vi "SetUp_Action.vi"(7 "Slot":T3, 8 "error in":errorcluster, 11 "GuiRef":T1={"StringOut"=refnum, "AbortOnFail"=refnum, "SN"=refnum, "SN_Length"=refnum, "TestResult"=refnum, "CycleTime"=refnum, "ErrorCode"=refnum, "UUTStatus"=refnum, "DataBaseEnable?"=refnum, "DUTModel"=refnum, "FixtureID"=refnum, "OperatorID"=refnum, "SNReady"=refnum, "StopSlot"=refnum, "NextStep"=refnum, "PassYeild"=refnum, "Failed"=refnum, "Passed"=refnum, "Tested"=refnum, "TestItemsCtl"={"StepName"="", "TestEnable"=FALSE, "LoopCount"=0, "StopOnFail"=FALSE, "Index"=0, "TestName"="", "通道"="", "参数"="", "TimeStart"=0}, "ProcessBar"=refnum, "Slot"=enum."Slot1", "Row"=3, "States"=refnum, "TestMode"=refnum, "循环次数-DUT"=refnum, "波形图"=refnum, "产品型号"=refnum, "子面板"=refnum, "测试失败项目"=refnum, "测试结果"=refnum, "DUT"=refnum, "Starttime"=refnum, "SlotReady"=refnum, "版本信息"=refnum, "WIFI_1"=refnum, "WIFI_2"=refnum, "直通率"=refnum, "卡1开卡结果"=refnum, "卡2开卡结果"=refnum}) -> (0 "error out":errorcluster, 3 "ScanSNOK":bool)   [LabVIEW 2013]
uses:
  SystemCode/SysControl/Slot.ctl
  SystemCode/SysControl/Reference.ctl
  SystemCode/SysControl/TestItemsCTL.ctl
  SystemCode/SysControl/LEDState.ctl
  GlobalValue.vi
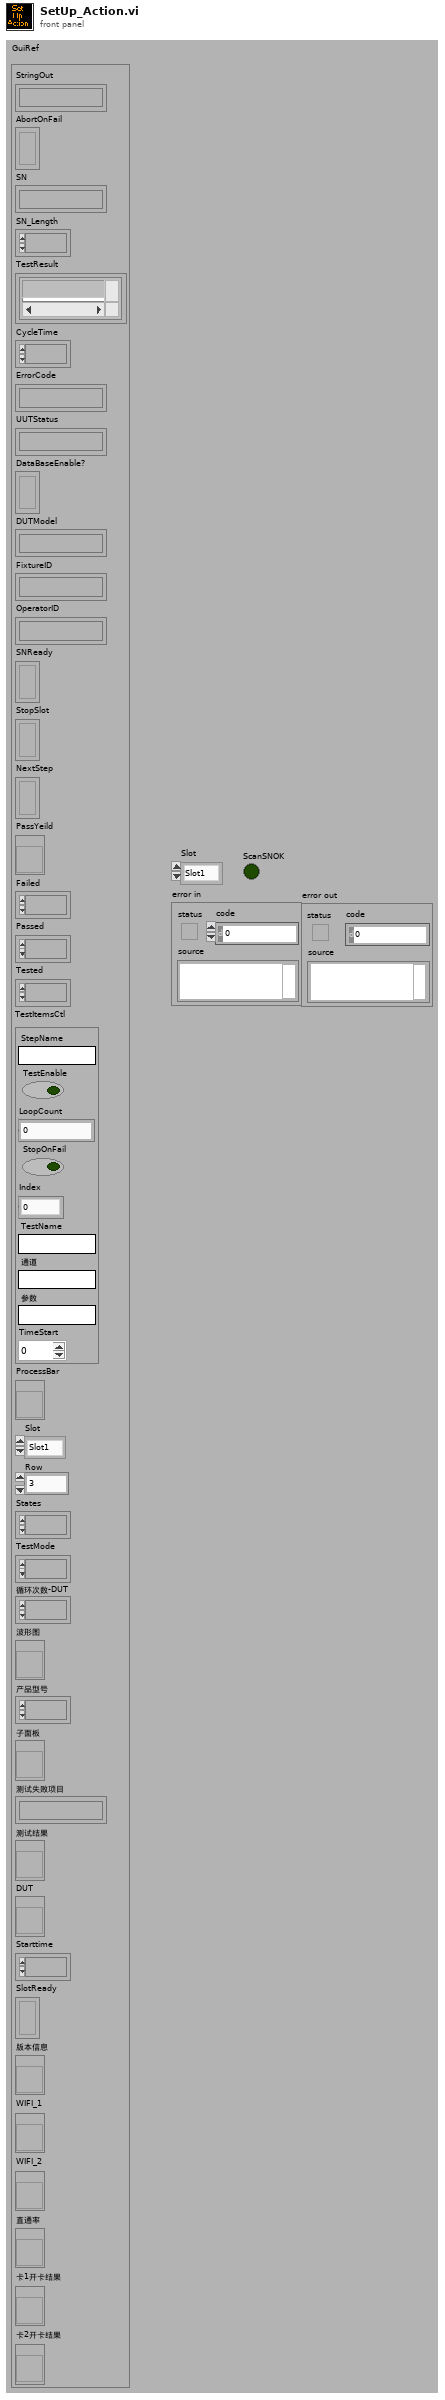
[diagram p1: front panel]
types:
  T1 = typedef "Reference.ctl" = cluster{"StringOut":refnum<vi>, "AbortOnFail":refnum<vi>, "SN":refnum<vi>, "SN_Length":refnum<vi>, "TestResult":refnum<vi>, "CycleTime":refnum<vi>, "ErrorCode":refnum<vi>, "UUTStatus":refnum<vi>, "DataBaseEnable?":refnum<vi>, "DUTModel":refnum<vi>, "FixtureID":refnum<vi>, "OperatorID":refnum<vi>, "SNReady":refnum<vi>, "StopSlot":refnum<vi>, "NextStep":refnum<vi>, "PassYeild":refnum<vi>, "Failed":refnum<vi>, "Passed":refnum<vi>, "Tested":refnum<vi>, "TestItemsCtl":T2, "ProcessBar":refnum<vi>, "Slot":T3, "Row":u32, "States":refnum<vi>, "TestMode":refnum<vi>, "循环次数-DUT":refnum<vi>, "波形图":refnum<vi>, "产品型号":refnum<vi>, "子面板":refnum<vi>, "测试失败项目":refnum<vi>, "测试结果":refnum<vi>, "DUT":refnum<vi>, "Starttime":refnum<vi>, "SlotReady":refnum<vi>, "版本信息":refnum<vi>, "WIFI_1":refnum<vi>, "WIFI_2":refnum<vi>, "直通率":refnum<vi>, "卡1开卡结果":refnum<vi>, "卡2开卡结果":refnum<vi>}
  T2 = typedef "TestItemsCTL.ctl" = cluster{"StepName":string, "TestEnable":bool, "LoopCount":i32, "StopOnFail":bool, "Index":u32, "TestName":string, "通道":string, "参数":string, "TimeStart":u32}
  T3 = typedef "Slot.ctl" = enum16{"Slot1", "Slot2", "Slot3", "Slot4"}
  T4 = typedef "LEDState.ctl" = enum16{"默认", "闪烁", "停止闪烁", "真", "假"}
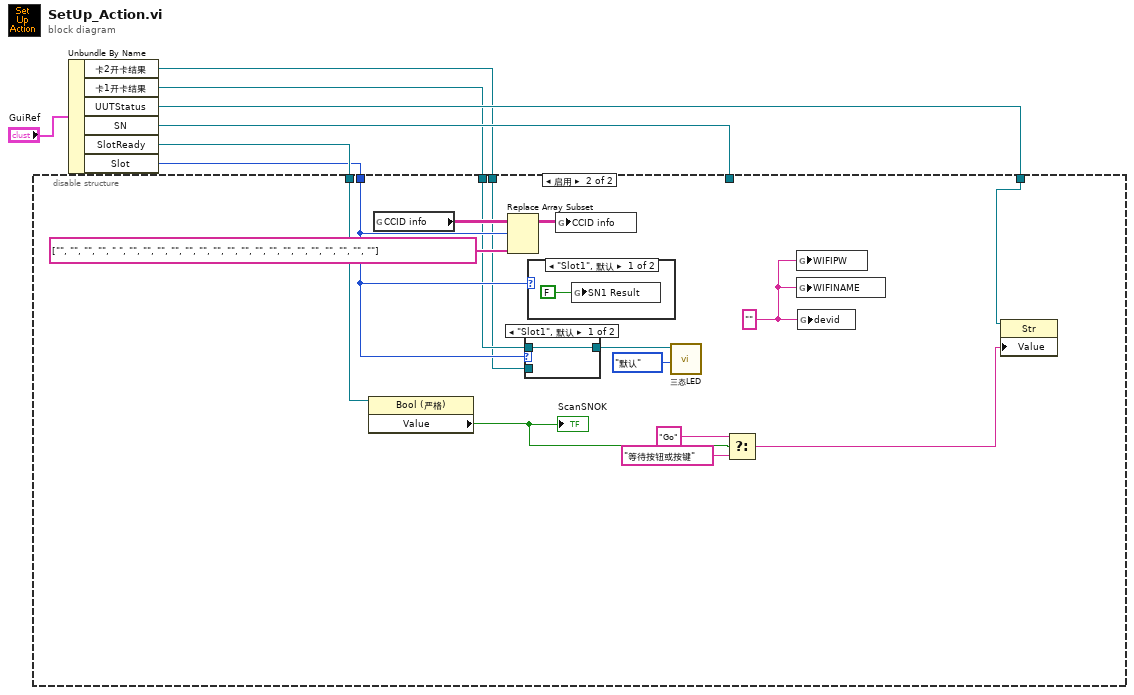
[diagram p0: block diagram]
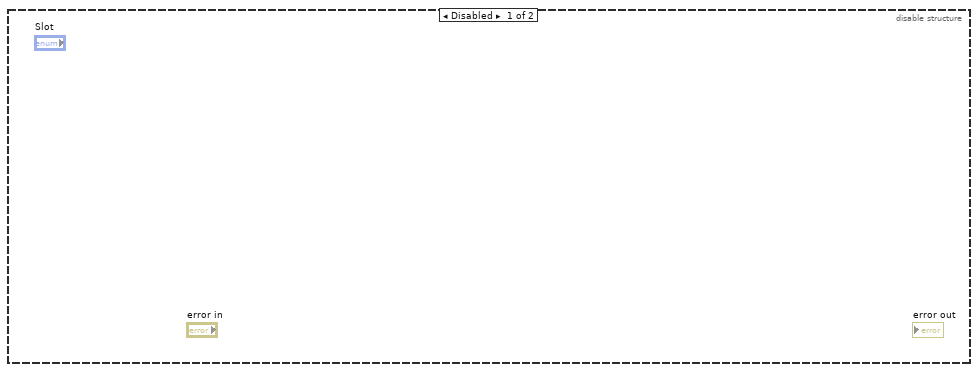
[diagram p2: hidden frame]
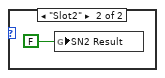
[diagram p4: hidden frame]
diagram:
  n1 = Unbundle By Name("GuiRef") -> ("卡2开卡结果"=w1:refnum<vi>, "卡1开卡结果"=w2:refnum<vi>, "UUTStatus"=w4:refnum<vi>, "SN"=w6:refnum<vi>, "SlotReady"=w5:refnum<vi>, "Slot"=w3:T3)
  n2 = disable-structure shown="启用" {
    disable-tunnel: w6 -> [_ _]
    disable-tunnel: w5 -> [_ w23]
    disable-tunnel: w4 -> [_ w22]
    disable-tunnel: w3 -> [_ w12]
    disable-tunnel: w2 -> [_ w11]
    disable-tunnel: w1 -> [_ w9]
    frame Disabled {
    }
    frame Enabled {
      w14 = "" ("devid")
      n3 = property class="Bool (严格)"(reference=w23) -> ("Value"=w21:bool)  [unwired: 1 in, 2 out]
      "ScanSNOK" <- w21
      n4 = global read "GlobalValue.vi" "CCID info"() -> (w17:string[][])
      n5 = Replace Array Subset(array=w17, new element=string[] ["", "", "", "", " ", "", "", "", "", "", "", "", "", "", "", "", "", "", "", "", "", "", ""], index (row)=w12) -> (w15:string[][])  [unwired: 1 in]
      n6 = case shown="\"Slot1\", 默认" w12 {
        tunnel: w11 -> [w24 _]
        tunnel: [w24 w25] -> w10
        tunnel: w9 -> [_ w25]
        frame "Slot1", Default {
        }
        frame "Slot2" {
        }
      }
      n7 = case shown="\"Slot1\", 默认" w12 {
        frame "Slot1", Default {
          n8 = global write "GlobalValue.vi" "SN1 Result"(FALSE ("SN Result")) -> ()
        }
        frame "Slot2" {
          n9 = global write "GlobalValue.vi" "SN2 Result"(FALSE ("SN Result")) -> ()
        }
      }
      n10 = global write "GlobalValue.vi" "CCID info"(w15) -> ()
      n11 = call "三态LED.vi"("State"=LEDState."默认", "Ctl引用句柄"=w10) -> ()  [unwired: 4 in, 2 out]
      n12 = Select(t="Go", s=w21, f="等待按钮或按键") -> (s? t:f=w18:string)
      n13 = global write "GlobalValue.vi" "WIFIPW"(w14) -> ()
      n14 = global write "GlobalValue.vi" "WIFINAME"(w14) -> ()
      n15 = global write "GlobalValue.vi" "devid"(w14) -> ()
      n16 = property class="Str"(reference=w22, "Value"=w18) -> ()  [unwired: 1 in, 2 out]
    }
  }
